vi "Export CmdResp Pair.vi"(8 "error in (no error)":errorcluster, 11 "Device Item Ref in":T1 format="%.0x") -> (0 "error out":errorcluster, 2 "Signals":T2 {"Response"."Byte Order" items=["Little Endian", "Big Endian"]; "Response"."Data Type" items=["Signed", "Unsigned", "IEEE Float"]; "Cmd"."Byte Order" items=["Little Endian", "Big Endian"]; "Cmd"."Data Type" items=["Signed", "Unsigned", "IEEE Float"]}, 3 "Section Ref out":T1 format="%.0x")   [LabVIEW 2015, in "Diagnostics Addon System Explorer.lvlib"]
uses:
  Diagnostics Addon System Explorer.lvlib
  Shared/Types/Command Response Signals.ctl
  Shared/Types/Signal Parameters.ctl
  <vilib>/NI Veristand/Custom Device API/Custom Device Item Ref.ctl
  Types/FG Action.ctl
  Signal Parameters FG.vi
  <vilib>/NI Veristand/Custom Device API/NI VeriStand - Get Item Property.vi
  <vilib>/NI Veristand/Custom Device API/Get Item Property (U32).vi
  <vilib>/NI Veristand/Custom Device API/NI VeriStand - Set Item Property.vi
  <vilib>/NI Veristand/Custom Device API/Set Item Property (U32).vi
  Shared/SubVIs/GUID Lookup.vi
  <vilib>/NI Veristand/Custom Device API/NI VeriStand - Get Custom Device Channel Data.vi
  <vilib>/NI Veristand/Custom Device API/NI VeriStand - Get Item Description.vi
  <vilib>/NI Veristand/Custom Device API/Get Item Property (String).vi
  <vilib>/NI Veristand/Custom Device API/Get Item Property (Double).vi
  <vilib>/NI Veristand/Custom Device API/Set Item Property (String).vi
  <vilib>/NI Veristand/Custom Device API/Set Item Property (Double).vi
  <vilib>/NI Veristand/Custom Device API/NI VeriStand - Get Item Children.vi
  <vilib>/NI Veristand/Custom Device Tools/Custom Device Utility Library/NI VeriStand - Search for Item by GUID.vi
  <vilib>/NI Veristand/Custom Device Tools/Custom Device Utility Library/Custom Device Utility Library.lvlib
  Shared/Diagnostics Addon Shared.lvlib
  <vilib>/NI Veristand/Custom Device API/Custom Device API.lvlib
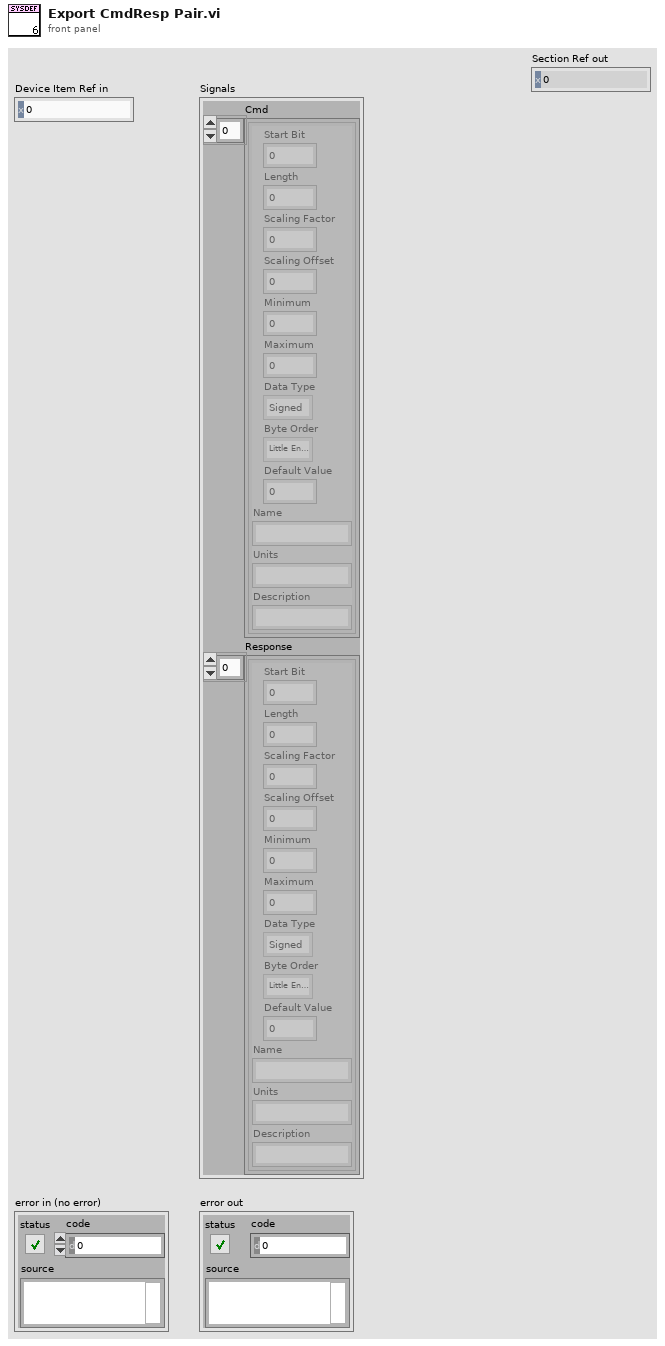
[diagram p1: front panel]
types:
  T1 = typedef "Custom Device API.lvlib/Custom Device Item Ref.ctl" = u64
  T2 = typedef "Diagnostics Addon Shared.lvlib/Command Response Signals.ctl" = cluster{"Cmd":T3[], "Response":T3[]}
  T3 = typedef "Diagnostics Addon Shared.lvlib/Signal Parameters.ctl" = cluster{"Start Bit":u8, "Length":u8, "Scaling Factor":dbl, "Scaling Offset":dbl, "Minimum":dbl, "Maximum":dbl, "Data Type":u32, "Byte Order":u32, "Default Value":dbl, "Name":string, "Units":string, "Description":string}
  T4 = typedef "Diagnostics Addon System Explorer.lvlib/FG Action.ctl" = enum16{"Get", "Set"}
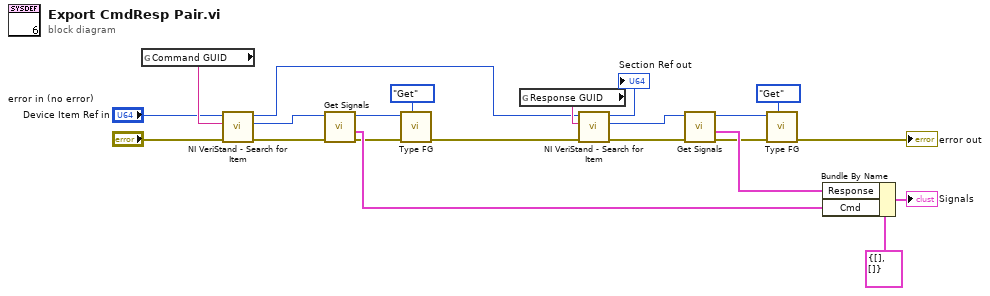
[diagram p0: block diagram]
diagram:
  n1 = global read "GUID Lookup.vi" "Command GUID"() -> (w13:string)
  n2 = call-poly <vilib>:"NI VeriStand - Search for Item.vi"("error in"="error in (no error)", "Item GUID"=w13, "Section Ref in"="Device Item Ref in") -> ("error out"=w15:errorcluster, "Item Ref"=w16:T1, "Section Ref out"=w9:T1)  [unwired: 5 in, 1 out]
  n3 = call "Get Signals.vi"("error in (no error)"=w15, "Device Item Ref out"=w16) -> ("error out"=w8:errorcluster, "Parameters"=w20:T3[], "Item Ref out"=w6:T1)  [unwired: 6 in, 1 out]
  n4 = call "Type FG.vi"("Action"=FG_Action."Get", "error in (no error)"=w8, "Device Item Ref in"=w6) -> ("error out"=w7:errorcluster)  [unwired: 6 in, 2 out]
  n5 = global read "GUID Lookup.vi" "Response GUID"() -> (w14:string)
  n6 = call-poly <vilib>:"NI VeriStand - Search for Item.vi"("error in"=w7, "Item GUID"=w14, "Section Ref in"=w9) -> ("error out"=w17:errorcluster, "Item Ref"=w18:T1, "Section Ref out"=→"Section Ref out":T1)  [unwired: 5 in, 1 out]
  n7 = call "Get Signals.vi"("error in (no error)"=w17, "Device Item Ref out"=w18) -> ("error out"=w3:errorcluster, "Parameters"=w21:T3[], "Item Ref out"=w1:T1)  [unwired: 6 in, 1 out]
  n8 = call "Type FG.vi"("Action"=FG_Action."Get", "error in (no error)"=w3, "Device Item Ref in"=w1) -> ("error out"=→"error out":errorcluster)  [unwired: 6 in, 2 out]
  n9 = Bundle By Name(cluster=T2 {"Cmd"=[], "Response"=[]} ("Signals"), "Response"=w21, "Cmd"=w20) -> (→"Signals":T2)
